vi "PantherScan File Path--constant.vi"(11 "Path":path) -> (3 "PantherScan file Path":path)   [LabVIEW 2019, in "Panther Dashboard.lvlib"]
uses:
  Panther Dashboard.lvlib
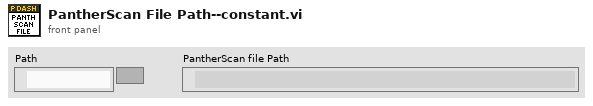
[diagram p1: front panel]
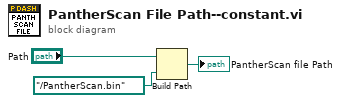
[diagram p0: block diagram]
diagram:
  n1 = Build Path(base path="Path", name or relative path=path "../PantherScan.bin") -> (appended path=→"PantherScan file Path":path)
